vi "Bluetooth.vi"() -> ()   [LabVIEW 2014]
panel:
  out "number of services":u16
  out "service list":T1(array[cluster])
  out "Address":string
  out "Device Name":string
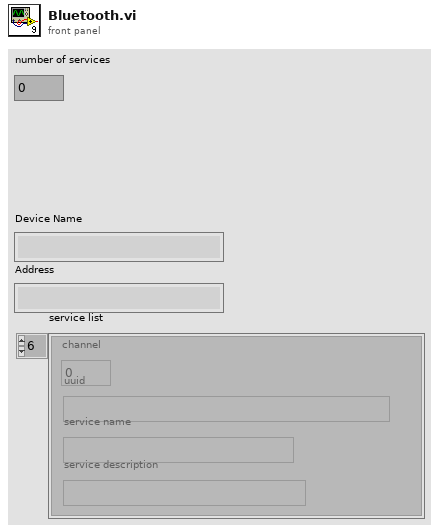
[diagram p1: front panel]
types:
  T1 = cluster{"channel":u16, "uuid":string, "service name":string, "service description":string}[]
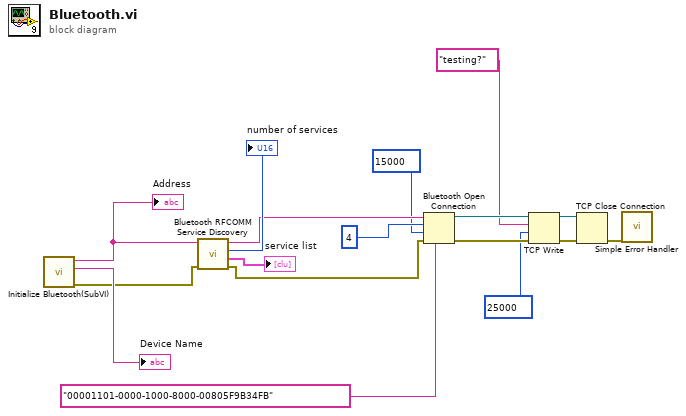
[diagram p0: block diagram]
diagram:
  n1 = call "Initialize Bluetooth(SubVI).vi"() -> ("error out"=w15:errorcluster, "Device Name"=→"Device Name":string, "Address"=w16:string)  [unwired: 9 in]
  "Address" <- w16
  n2 = call <vilib>:"Bluetooth RFCOMM Service Discovery.vi"("error in (no error)"=w15, "address in"=w16) -> ("error out"=w9:errorcluster, "service list"=→"service list":T1, "number of services"=→"number of services":u16, "address out"=w12:string)  [unwired: 2 in]
  n3 = Bluetooth Open Connection(6:"00001101-0000-1000-8000-00805F9B34FB" ("uuid"), 8:w9, 9:15000 ("timeout ms (60000)"), 10:u16 4 ("channel (0)"), 11:w12) -> (0:w6:errorcluster, 3:w7:refnum<k31>)
  n4 = TCP Write(connection ID=w7, data in="testing?", error in (no error)=w6, 9:25000 ("timeout ms (25000)")) -> (connection ID out=w3:refnum<k31>, error out=w2:errorcluster)  [unwired: 1 out]
  n5 = TCP Close Connection(connection ID=w3, error in (no error)=w2) -> (error out=w1:errorcluster)  [unwired: 1 in, 1 out]
  n6 = call <vilib>:"Simple Error Handler.vi"("error in (no error)"=w1) -> ()  [unwired: 4 in, 5 out]
